vi "GetParentQualifiedName.vi"(8 "error in (no error)":errorcluster, 11 "CLabVIEWItem in":refnum<class "CLabVIEWItem.lvclass">) -> (0 "error out":errorcluster, 1 "Name":string, 3 "CLabVIEWItem out":refnum<class "CLabVIEWItem.lvclass">)   [LabVIEW 2020, in "LabVIEWItem.lvlib" / "CLabVIEWItem.lvclass"]
uses:
  CLabVIEWItem.lvclass
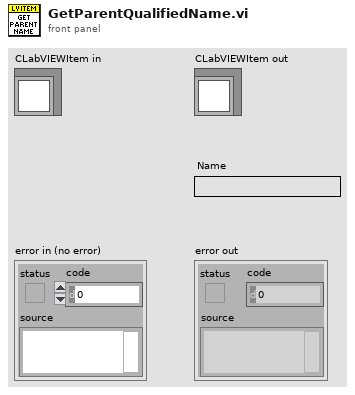
[diagram p1: front panel]
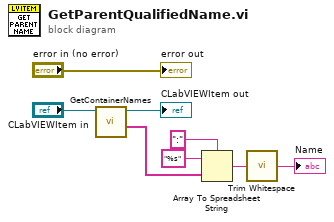
[diagram p0: block diagram]
diagram:
  n1 = call-dynamic "GetContainerNames.vi"("CLabVIEWItem in"="CLabVIEWItem in") -> ("Container name[]"=w4:string[], "CLabVIEWItem out"=→"CLabVIEWItem out":refnum<class "CLabVIEWItem.lvclass">)  [unwired: 8 in, 1 out]
  n2 = Array To Spreadsheet String(delimiter (Tab)=":", array=w4, 3:"%s" ("format string")) -> (spreadsheet string=w5:string)
  n3 = call <vilib>:"Trim Whitespace.vi"("string"=w5) -> ("trimmed string"=→"Name":string)  [unwired: 1 in]
  "error out" <- "error in (no error)"
